vi "VNA Measurement Parameters Constructor2.vi"(0 "P1 Ref Plane Ext Time":dbl, 1 "P2 Ref Plane Ext Time":dbl, 2 "Sweep Frequency Start":dbl, 3 "Port 1 Correction Factors":cdb[][](array[numeric]), 4 "Port 2 Correction Factors":cdb[][](array[numeric]), 5 "Averaging Count":i32, 8 "Instrument Session":string) -> (7 "VNA Measurement Parameters Out":T1)   [LabVIEW 2013]
uses:
  VNA Measurement Parameters2.ctl
panel:
  in  "VNA Measurement Parameters":T1
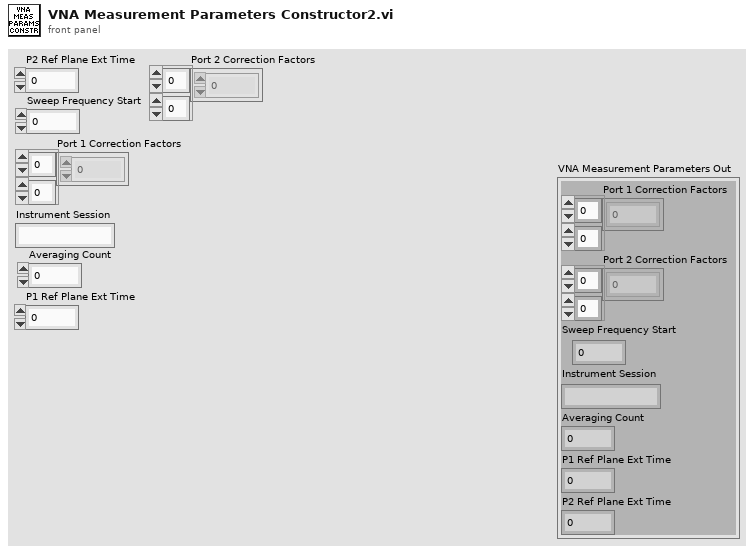
[diagram p1: front panel]
types:
  T1 = typedef "VNA Measurement Parameters2.ctl" = cluster{"Port 1 Correction Factors":cdb[][], "Port 2 Correction Factors":cdb[][], "Sweep Frequency Start":dbl, "Instrument Session":string, "Averaging Count":i32, "P1 Ref Plane Ext Time":dbl, "P2 Ref Plane Ext Time":dbl}
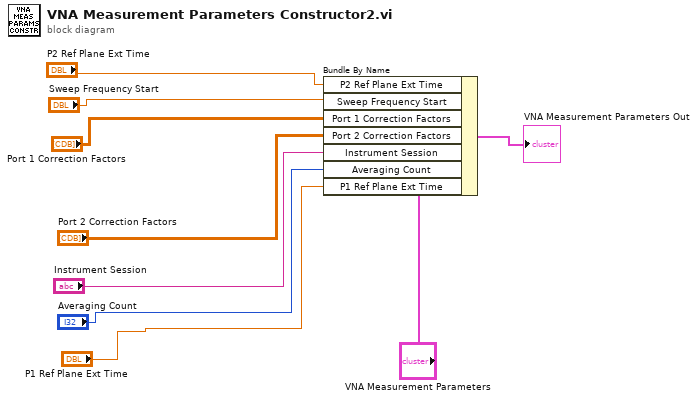
[diagram p0: block diagram]
diagram:
  n1 = Bundle By Name(cluster="VNA Measurement Parameters", "P2 Ref Plane Ext Time"="P2 Ref Plane Ext Time", "Sweep Frequency Start"="Sweep Frequency Start", "Port 1 Correction Factors"="Port 1 Correction Factors", "Port 2 Correction Factors"="Port 2 Correction Factors", "Instrument Session"="Instrument Session", "Averaging Count"="Averaging Count", "P1 Ref Plane Ext Time"="P1 Ref Plane Ext Time") -> (→"VNA Measurement Parameters Out":T1)
